vi "log_motor_moves_correction.vi"(6 "Motor Adress":T1(ring)=enum."3", 7 "waypoint version":bool, 8 "error in":errorcluster, 9 "Direction":i32, 10 "Log File IN":string, 11 "Delta Steps":i32) -> (0 "error out":errorcluster, 2 "Log File OUT":string)   [LabVIEW 2013]
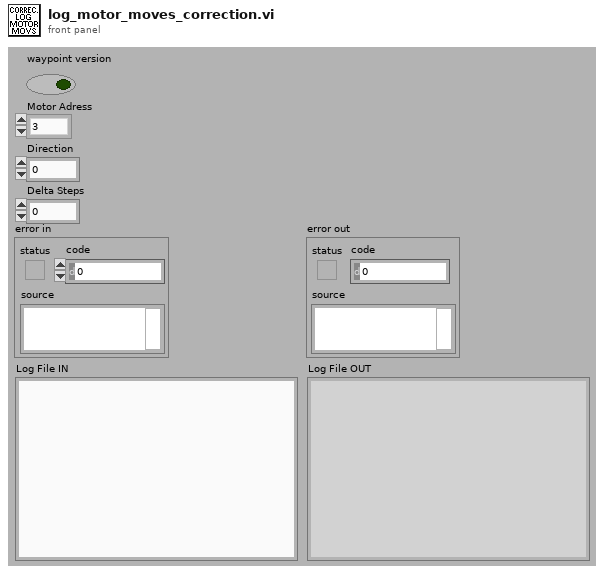
[diagram p1: front panel]
types:
  T1 = enum16{"All", "1", "2", "3", "4", "5", "6", "7", "8"}
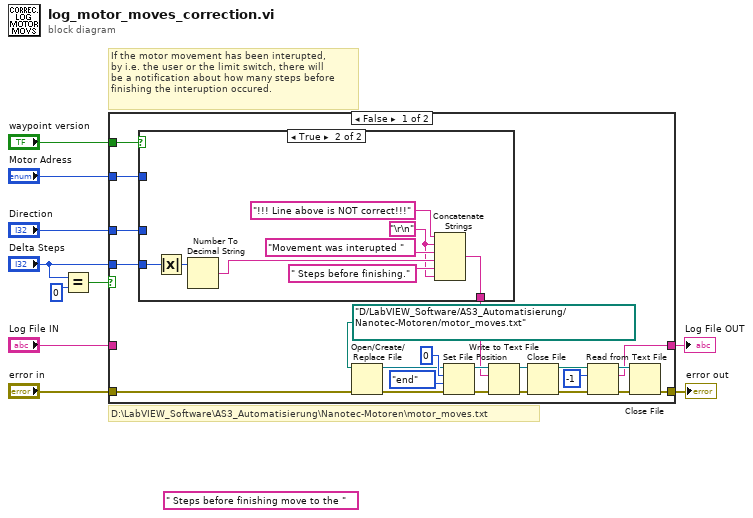
[diagram p0: block diagram]
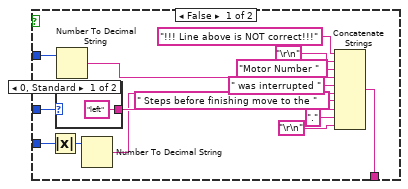
[diagram p2: hidden frame]
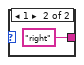
[diagram p3: hidden frame]
diagram:
  (unwired) " Steps before finishing move to the " ("string")
  # "D:\\LabVIEW_Software\\AS3_Automatisierung\\Nanotec-Motoren\\motor_moves.txt"
  # "If the motor movement has been interupted,\nby i.e. the user or the limit switch, there will\nbe a notification about how many steps before\nfinishing the interuption occured."
  n1 = Equal?(x="Delta Steps", y=u32 0) -> (x = y?=w10:bool)
  n2 = case shown="False" w10 {
    tunnel: [w14 w59] -> w9
    tunnel: [w17 w58] -> w8
    tunnel: "Log File IN" -> [_ w59]
    tunnel: "error in" -> [w15 w58]
    tunnel: "Direction" -> [w16 _]
    tunnel: "Delta Steps" -> [w12 _]
    tunnel: "Motor Adress" -> [w13 _]
    tunnel: "waypoint version" -> [w11 _]
    frame False {
      n3 = case shown="True" w11 {
        tunnel: [w45 w56] -> w18
        tunnel: w16 -> [w42 _]
        tunnel: w13 -> [w40 _]
        tunnel: w12 -> [w36 w55]
        frame False {
          n4 = Absolute Value(x=w36) -> (abs(x)=w35:i32)
          n5 = case shown="0, Standard" w42 {
            tunnel: ["left" "right"] -> w41
            frame 0, Default {
            }
            frame 1 {
            }
          }
          n6 = Number To Decimal String(number=w40) -> (decimal integer string=w39:string)  [unwired: 1 in]
          n7 = Number To Decimal String(number=w35) -> (decimal integer string=w38:string)  [unwired: 1 in]
          n8 = Concatenate Strings("!!! Line above is NOT correct!!!" ("string"), "\r\n", "Motor Number " ("string"), w39, " was interrupted " ("string"), w38, " Steps before finishing move to the " ("string"), w41, "." ("string"), "\r\n") -> (w45:string)
        }
        frame True {
          w50 = "\r\n"
          n9 = Absolute Value(x=w55) -> (abs(x)=w54:i32)
          n10 = Number To Decimal String(number=w54) -> (decimal integer string=w52:string)  [unwired: 1 in]
          n11 = Concatenate Strings("!!! Line above is NOT correct!!!" ("string"), w50, "Movement was interupted " ("string"), w52, " Steps before finishing." ("string"), w50) -> (w56:string)
        }
      }
      n12 = Open/Create/Replace File(file path (use dialog)=path "D:/LabVIEW_Software/AS3_Automatisierung/Nanotec-Motoren/motor_moves.txt", error in=w15) -> (refnum out=w27:refnum<file>, error out=w28:errorcluster)  [unwired: 4 in, 1 out]
      n13 = Set File Position(offset (in bytes) (0)=i64 0, refnum=w27, from (0:start)=enum16{"start", "end", "current"}."end", error in=w28) -> (refnum out=w29:refnum<file>, error out=w30:errorcluster)
      n14 = Write to Text File(file (use dialog)=w29, text=w18, error in=w30) -> (refnum out=w23:refnum<file>, error out=w24:errorcluster)  [unwired: 1 in, 1 out]
      n15 = Close File(refnum=w23, error in=w24) -> (path=w25:path, error out=w26:errorcluster)
      n16 = Read from Text File(file (use dialog)=w25, count=-1, error in=w26) -> (refnum out=w20:refnum<file>, text=w14:string, error out=w21:errorcluster)  [unwired: 1 in, 1 out]
      n17 = Close File(refnum=w20, error in=w21) -> (error out=w17:errorcluster)  [unwired: 1 out]
    }
    frame True {
    }
  }
  "error out" <- w8
  "Log File OUT" <- w9
